vi "Check Accessibility.vi"(7 "Error if denied? (F)":bool, 8 "error in (no error)":errorcluster, 11 "SMO in":refnum<class "SMO.lvclass">) -> (0 "error out":errorcluster, 1 "Accessible":bool, 3 "SMO out":refnum<class "SMO.lvclass">)   [LabVIEW 2013, in "SMO.lvclass"]
uses:
  SMO.lvclass
  SMO.lvclass/SMO.ctl
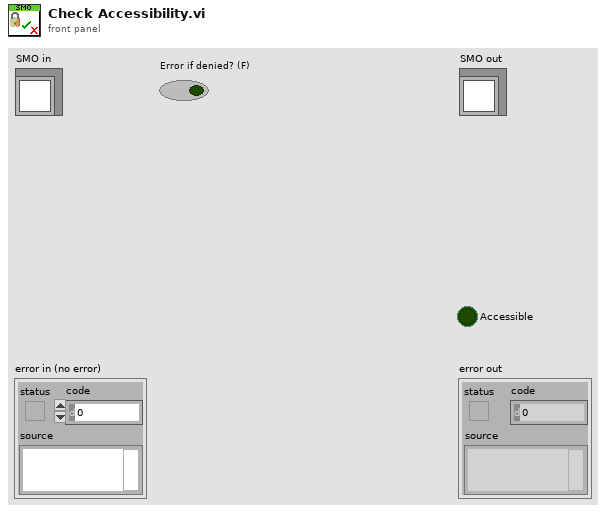
[diagram p1: front panel]
types:
  T1 = typedef "SMO.lvclass/Reserve State--Enum.ctl" = enum16{"Unreserved", "Reserved", "Self-locked"}
  T2 = typedef "SMO.lvclass/Accessibility--Cluster.ctl" = cluster{"Lock Key":string, "Reserve State":T1}
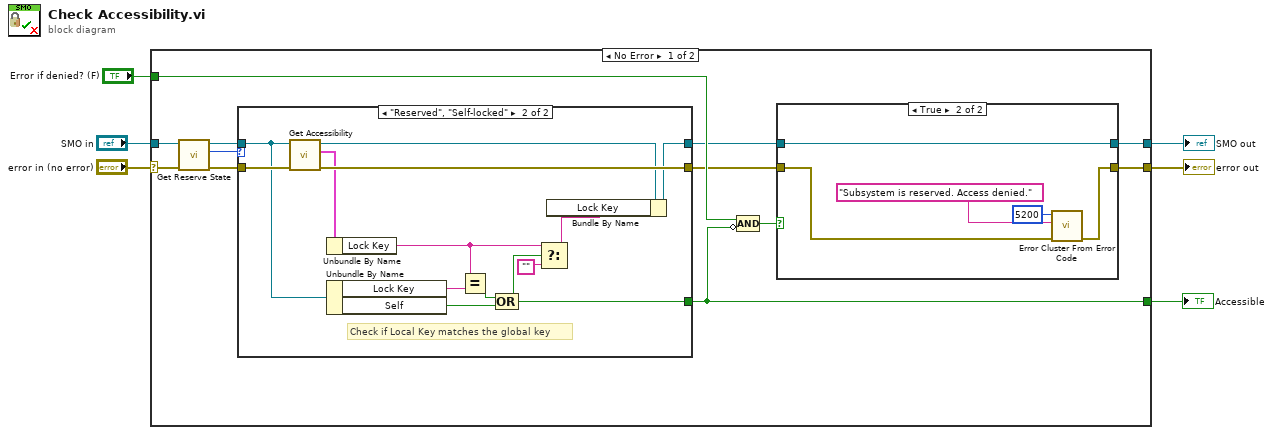
[diagram p0: block diagram]
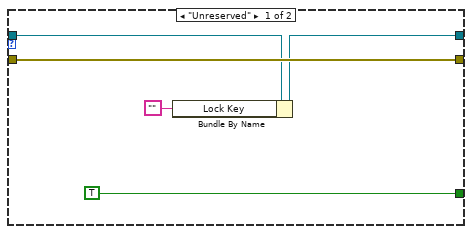
[diagram p3: hidden frame]
diagram:
  n1 = case shown="No Error" "error in (no error)" {
    selector: "error in (no error)" -> [w17 w45]
    tunnel: [w8 w45] -> w5
    tunnel: [w10 w44] -> w3
    tunnel: "SMO in" -> [w18 w44]
    tunnel: [w13 _] -> w2
    tunnel: "Error if denied? (F)" -> [w12 _]
    frame No Error {
      n2 = call "Get Reserve State.vi"("error in (no error)"=w17, "SMO"=w18) -> ("error out"=w16:errorcluster, "Reserve State"=w14:T1, "SMO out"=w15:refnum<class "SMO.lvclass">)  [unwired: 7 in]
      n3 = case shown="\"Reserved\", \"Self-locked\"" w14 {
        tunnel: w16 -> [w30 w43]
        tunnel: w15 -> [w27 w40]
        tunnel: [w26 w32] -> w9
        tunnel: [w30 w42] -> w7
        tunnel: [TRUE w35] -> w13
        frame "Unreserved" {
          n4 = Bundle By Name(cluster=w27, "Lock Key"="") -> (w26:refnum<class "SMO.lvclass">)
        }
        frame "Reserved", "Self-locked" {
          # "Check if Local Key matches the global key"
          n5 = call "Get Accessibility.vi"("error in (no error)"=w43, "SMO"=w40) -> ("error out"=w42:errorcluster, "Accessibility"=w41:T2, "SMO out"=w33:refnum<class "SMO.lvclass">)  [unwired: 7 in]
          n6 = Unbundle By Name(w41) -> ("Lock Key"=w36:string)
          n7 = Unbundle By Name(w40) -> ("Lock Key"=w39:string, "Self"=w38:bool)
          n8 = Equal?(x=w36, y=w39) -> (x = y?=w37:bool)
          n9 = Compound Arithmetic op=OR(w37, w38) -> (w35:bool)
          n10 = Select(t=w36, s=w35, f="") -> (s? t:f=w34:string)
          n11 = Bundle By Name(cluster=w33, "Lock Key"=w34) -> (w32:refnum<class "SMO.lvclass">)
        }
      }
      n12 = Compound Arithmetic op=AND(w12, invert w13) -> (w11:bool)
      n13 = case shown="True" w11 {
        tunnel: [w20 w25] -> w10
        tunnel: w9 -> [w20 w25]
        tunnel: w7 -> [w19 w24]
        tunnel: [w19 w23] -> w8
        frame False {
        }
        frame True {
          n14 = call <vilib>:"Error Cluster From Error Code.vi"("error in (no error)"=w24, "error message (\"\")"="Subsystem is reserved. Access denied.", "error code (0)"=5200) -> ("error out"=w23:errorcluster)  [unwired: 6 in]
        }
      }
    }
    frame Error {
    }
  }
  "error out" <- w5
  "SMO out" <- w3
  "Accessible" <- w2
